vi "QCA Get Channel Names.vi"() -> (0 "Channel Names":string[](array[string]))   [LabVIEW 2009]
uses:
  QCA Global.vi
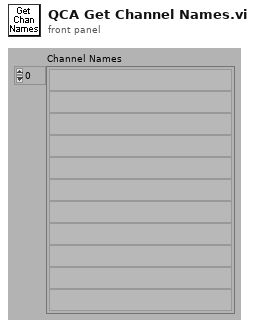
[diagram p1: front panel]
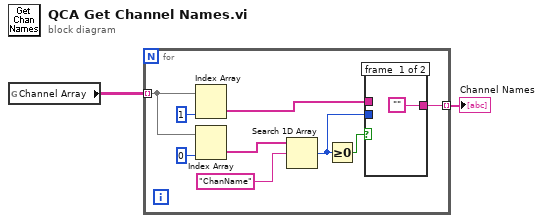
[diagram p0: block diagram]
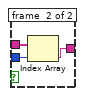
[diagram p2: hidden frame]
diagram:
  n1 = global read "QCA Global.vi" "Channel Array"() -> (w2:string[][][])
  n2 = for {
    tunnel: w2 -> [w9] mode=indexing
    tunnel: [w5] -> w1 mode=indexing
    n3 = Index Array(array=w9, index (col)=1 ("Index")) -> (element=w6:string[])  [unwired: 1 in]
    n4 = Index Array(array=w9, index (col)=0 ("Index")) -> (element=w8:string[])  [unwired: 1 in]
    n5 = Search 1D Array(1D array=w8, element="ChanName") -> (index of element=w4:i32)  [unwired: 1 in]
    n6 = Greater Or Equal To 0?(x=w4) -> (x >= 0?=w3:bool)
    n7 = case shown="True" w3 {
      tunnel: w6 -> [_ w15]
      tunnel: w4 -> [_ w14]
      tunnel: ["" w13] -> w5
      frame #0 {
      }
      frame #1 {
        n8 = Index Array(array=w15, index=w14) -> (element=w13:string)
      }
    }
  }
  "Channel Names" <- w1
